vi "Autosize Clusters.vi"(6 "Variant in":variant, 7 "Shift Pressed?":bool, 8 "error in (no error)":errorcluster, 10 "QD Combo Box Ref":refnum<vi>, 11 "QD Launch VI Ref":refnum<vi>) -> (0 "error out":errorcluster, 4 "Variant out":variant)   [LabVIEW 2013]
doc: "Changes the autosize property of all selected clusters. This works on both front panel and block diagram.\nBy default the autosizing is set to \"Arrange Vertically\". The following input changes this behaviour :\n\nNone : \"None\"\nSize to Fit : \"Auto\", \"Fit\", \"Size to Fit\"\nArrange Horizontally : \"Arrange Horizontally\", \"H\", \"Hor\", \"Horizontally\"\nArrange Vertically : \"Arrange Vertically\", \"V\", \"Vert\", \"Vertically\"\n\nDefault Shortcut - [Z]"
panel:
  in  "Undo Name":string="Change Cluster Autosizing"
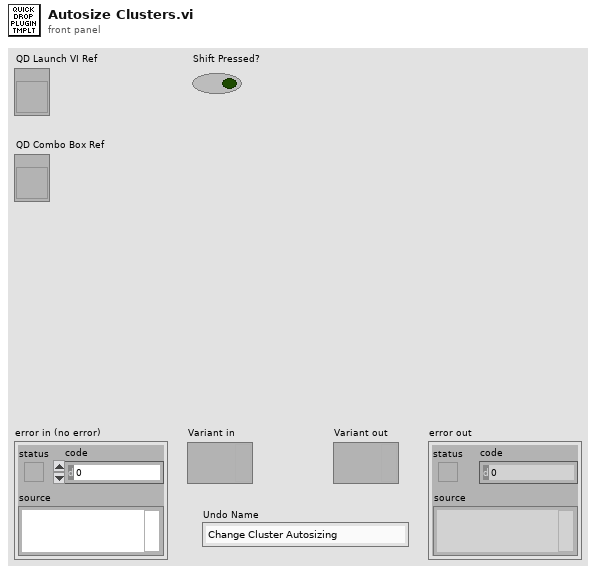
[diagram p1: front panel]
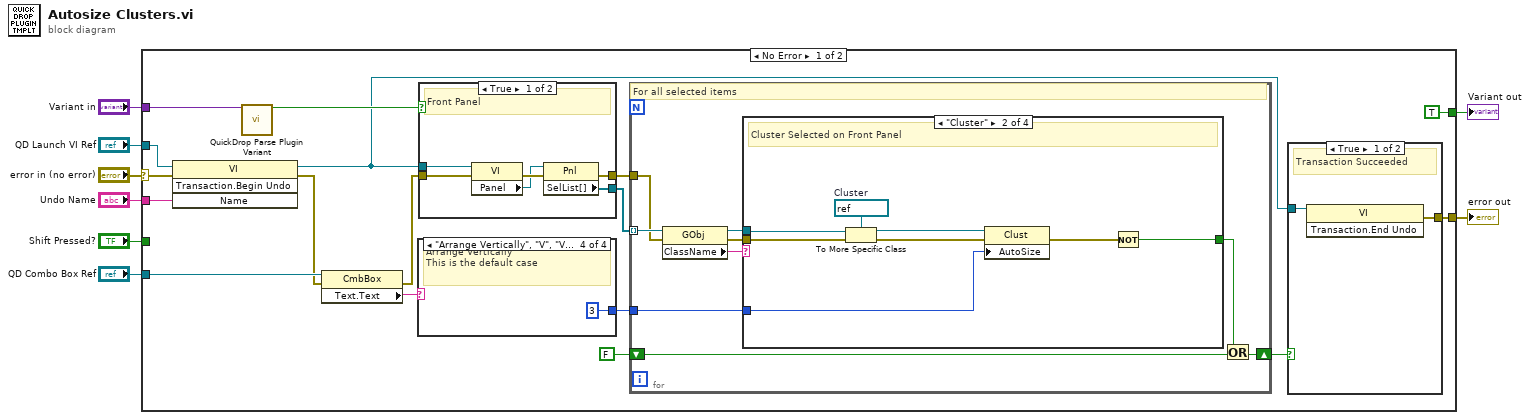
[diagram p0: block diagram]
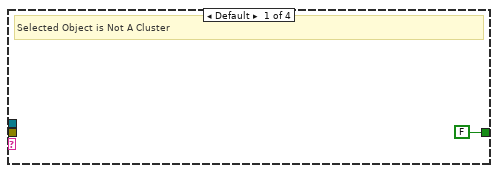
[diagram p2: hidden frame]
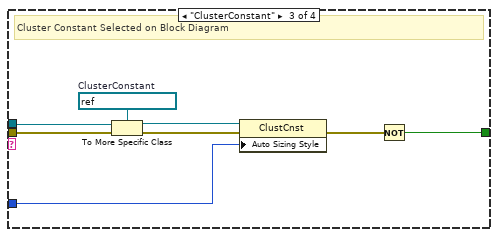
[diagram p3: hidden frame]
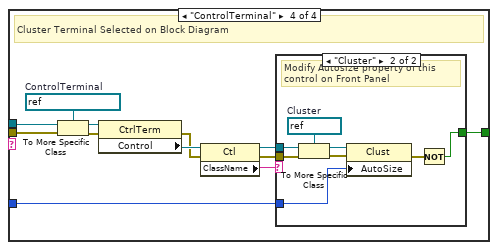
[diagram p4: hidden frame]
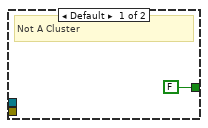
[diagram p5: hidden frame]
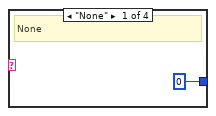
[diagram p6: hidden frame]
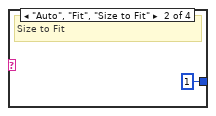
[diagram p7: hidden frame]
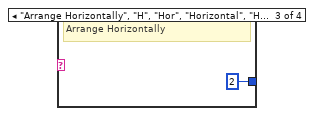
[diagram p8: hidden frame]
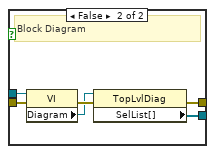
[diagram p9: hidden frame]
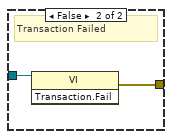
[diagram p10: hidden frame]
diagram:
  n1 = case shown="No Error" "error in (no error)" {
    selector: "error in (no error)" -> [w24 w93]
    tunnel: [w21 w93] -> w7
    tunnel: "QD Launch VI Ref" -> [w11 _]
    tunnel: "Shift Pressed?" -> [_ _]
    tunnel: "QD Combo Box Ref" -> [w16 _]
    tunnel: "Variant in" -> [w25 _]
    tunnel: "Undo Name" -> [w9 _]
    tunnel: [TRUE _] -> w1
    frame No Error {
      n2 = invoke class="VI" method="Transaction.Begin Undo"(reference=w11, error in=w24, "Name"=w9) -> (reference out=w10:refnum<vi>, error out=w13:errorcluster)  [unwired: 1 in, 2 out]
      n3 = call <vilib>:"QuickDrop Parse Plugin Variant.vi"("QDKS Variant in"=w25) -> ("QD Launch VI Panel?"=w22:bool)  [unwired: 12 in, 2 out]
      n4 = property class="CmbBox"(reference=w16, error in=w13) -> (error out=w12:errorcluster, "Text.Text"=w15:string)  [unwired: 1 out]
      n5 = case shown="\"Arrange Vertically\", \"V\", \"Vertical\", \"Vertically\", Default" w15 {
        tunnel: [u32 0 ("Auto Sizing") u32 1 ("Auto Sizing") u32 2 ("Auto Sizing") u32 3 ("Auto Sizing")] -> w14
        frame "None" {
          # "None"
        }
        frame "Auto", "Fit", "Size to Fit" {
          # "Size to Fit"
        }
        frame "Arrange Horizontally", "H", "Hor", "Horizontal", "Horizontally" {
          # "Arrange Horizontally"
        }
        frame "Arrange Vertically", "V", "Vertical", "Vertically", Default {
          # "Arrange Vertically\nThis is the default case"
        }
      }
      n6 = case shown="True" w22 {
        tunnel: w12 -> [w82 w88]
        tunnel: w10 -> [w81 w87]
        tunnel: [w77 w83] -> w20
        tunnel: [w78 w84] -> w17
        frame True {
          # "Front Panel"
          n7 = property class="VI"(reference=w81, error in=w82) -> (error out=w80:errorcluster, "Panel"=w79:refnum<vi>)  [unwired: 1 out]
          n8 = property class="Pnl"(reference=w79, error in=w80) -> (error out=w77:errorcluster, "SelList[]"=w78:refnum<vi>[])  [unwired: 1 out]
        }
        frame False {
          # "Block Diagram"
          n9 = property class="VI"(reference=w87, error in=w88) -> (error out=w86:errorcluster, "Diagram"=w85:refnum<vi>)  [unwired: 1 out]
          n10 = property class="TopLvlDiag"(reference=w85, error in=w86) -> (error out=w83:errorcluster, "SelList[]"=w84:refnum<vi>[])  [unwired: 1 out]
        }
      }
      n11 = for {
        shift-right: [w26] -> w18
        shift-left: FALSE -> [w31]
        tunnel: w17 -> [w34] mode=indexing
        tunnel: w20 -> [w28]
        tunnel: w14 -> [w29]
        # "For all selected items"
        n12 = property class="GObj"(reference=w34, error in=w28) -> (reference out=w33:refnum<vi>, error out=w32:errorcluster, "ClassName"=w27:string)
        n13 = case shown="\"Cluster\"" w27 {
          tunnel: w33 -> [_ w41 w49 w61]
          tunnel: w32 -> [_ w42 w50 w62]
          tunnel: [FALSE w39 w47 w60] -> w30
          tunnel: w29 -> [_ w37 w44 w59]
          frame Default {
            # "Selected Object is Not A Cluster"
          }
          frame "Cluster" {
            w43 = refnum<vi> refnum  # Cluster
            # "Cluster Selected on Front Panel"
            n14 = To More Specific Class(target class=w43, reference=w41, error in=w42) -> (specific class reference=w38:refnum<vi>, error out=w40:errorcluster)
            n15 = property class="Clust"(reference=w38, error in=w40, "AutoSize"=w37) -> (error out=w36:errorcluster)  [unwired: 1 out]
            n16 = Not(x=w36) -> (.not. x?=w39:bool)
          }
          frame "ClusterConstant" {
            w51 = refnum<vi> refnum  # ClusterConstant
            # "Cluster Constant Selected on Block Diagram"
            n17 = To More Specific Class(target class=w51, reference=w49, error in=w50) -> (specific class reference=w46:refnum<vi>, error out=w48:errorcluster)
            n18 = property class="ClustCnst"(reference=w46, error in=w48, "Auto Sizing Style"=w44) -> (error out=w45:errorcluster)  [unwired: 1 out]
            n19 = Not(x=w45) -> (.not. x?=w47:bool)
          }
          frame "ControlTerminal" {
            w63 = refnum<vi> refnum  # ControlTerminal
            # "Cluster Terminal Selected on Block Diagram"
            n20 = To More Specific Class(target class=w63, reference=w61, error in=w62) -> (specific class reference=w58:refnum<vi>, error out=w52:errorcluster)
            n21 = property class="CtrlTerm"(reference=w58, error in=w52) -> (error out=w56:errorcluster, "Control"=w57:refnum<vi>)  [unwired: 1 out]
            n22 = property class="Ctl"(reference=w57, error in=w56) -> (reference out=w53:refnum<vi>, error out=w54:errorcluster, "ClassName"=w55:string)
            n23 = case shown="\"Cluster\"" w55 {
              tunnel: [FALSE w72] -> w60
              tunnel: w59 -> [_ w71]
              tunnel: w54 -> [_ w68]
              tunnel: w53 -> [_ w69]
              frame Default {
                # "Not A Cluster"
              }
              frame "Cluster" {
                w70 = refnum<vi> refnum  # Cluster
                # "Modify Autosize property of this control on Front Panel"
                n24 = To More Specific Class(target class=w70, reference=w69, error in=w68) -> (specific class reference=w67:refnum<vi>, error out=w66:errorcluster)
                n25 = property class="Clust"(reference=w67, error in=w66, "AutoSize"=w71) -> (error out=w65:errorcluster)  [unwired: 1 out]
                n26 = Not(x=w65) -> (.not. x?=w72:bool)
              }
            }
          }
        }
        n27 = Or(x=w30, y=w31) -> (x .or. y?=w26:bool)
      }
      n28 = case shown="True" w18 {
        tunnel: w10 -> [w89 w91]
        tunnel: [w90 w92] -> w21
        frame True {
          # "Transaction Succeeded"
          n29 = invoke class="VI" method="Transaction.End Undo"(reference=w89) -> (error out=w90:errorcluster)  [unwired: 2 in, 2 out]
        }
        frame False {
          # "Transaction Failed"
          n30 = invoke class="VI" method="Transaction.Fail"(reference=w91) -> (error out=w92:errorcluster)  [unwired: 2 in, 2 out]
        }
      }
    }
    frame Error {
    }
  }
  "error out" <- w7
  "Variant out" <- w1
